vi "Write Data Type.vi"(8 "error in (no error)":errorcluster, 10 "data type":T1, 11 "Update Tag in":refnum<class "Update Tag.lvclass">) -> (0 "error out":errorcluster, 3 "Update Tag out":refnum<class "Update Tag.lvclass">)   [LabVIEW 2015, in "Update Tag.lvclass"]
uses:
  Update Tag.lvclass
  <vilib>/NI/Tag Bus/tag/Data Type.ctl
  Update Tag.lvclass/Update Tag.ctl
  <vilib>/NI/Tag Bus/tag/tag descriptor.lvclass
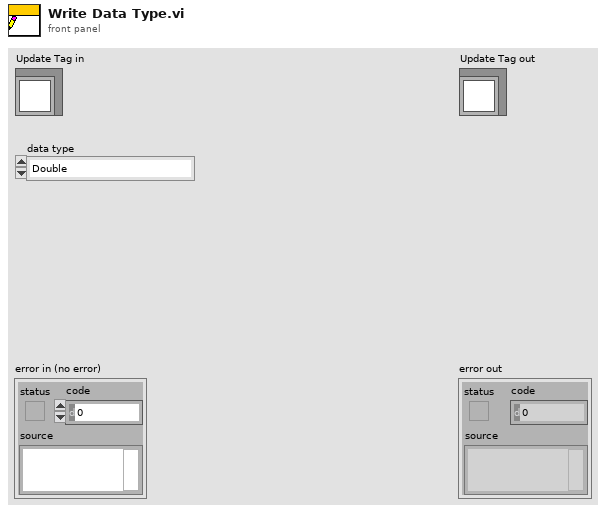
[diagram p1: front panel]
types:
  T1 = typedef "tag bus.lvlib/tag descriptor.lvclass/Data Type.ctl" = enum16{"Double", "Single", "I64", "I32", "I16", "I8", "U64", "U32", "U16", "U8", "Boolean", "String", "Array of Double", "Array of Single", "Array of I64", "Array of I32", "Array of I16", "Array of I8", "Array of U64", "Array of U32", "Array of U16", "Array of U8", "Array of Boolean", "Array of String"}
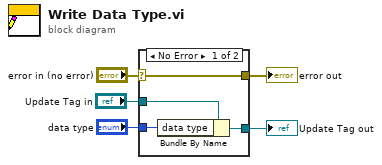
[diagram p0: block diagram]
diagram:
  n1 = case shown="No Error" "error in (no error)" {
    selector: "error in (no error)" -> [w9 w10]
    tunnel: [w9 w10] -> w4
    tunnel: [w7 w11] -> w2
    tunnel: "Update Tag in" -> [w8 w11]
    tunnel: "data type" -> [w6 _]
    frame No Error {
      n2 = Bundle By Name(cluster=w8, "data type"=w6) -> (w7:refnum<class "Update Tag.lvclass">)
    }
    frame Error {
    }
  }
  "error out" <- w4
  "Update Tag out" <- w2
